vi "pulse data selector.vi"(0 "file path (dialog if empty)":path, 9 "y axis":u16(ring)=3 items=["time", "rate of change of B", "magnetic field", "signal A", "signal B", "1/B"]) -> (5 "file path":path, 6 "1/B start interpolation":dbl format="%.2f", 8 "1/B end interpolation":dbl format="%.2f", 10 "time rising":dbl[](array[numeric]) format="%.2f", 11 "ch B falling":dbl[](array[numeric]) format="%.2f", 12 "time falling":dbl[](array[numeric]) format="%.2f", 13 "ch B rising":dbl[](array[numeric]) format="%.2f", 14 "dB/dt rising":dbl[](array[numeric]) format="%.2f", 15 "dB/dt falling":dbl[](array[numeric]) format="%.2f", 16 "B rising":dbl[](array[numeric]) format="%.2f", 17 "B falling":dbl[](array[numeric]) format="%.2f", 18 "ch A rising":dbl[](array[numeric]) format="%.2f", 19 "ch A falling":dbl[](array[numeric]) format="%.2f")   [LabVIEW 2016]
uses:
  <vilib>/Utility/file.llb/Read From Spreadsheet File (DBL).vi
  <vilib>/Analysis/NI_AALPro.lvlib
panel:
  in  "subtract reference trace? copy 2":bool
  in  "mult fac.":dbl=1.0 format="%.2f"
  in  "subtract reference trace? copy":bool
  in  "with dB/dt":bool
  in  "background":u16(ring) items=["subtract fitted background", "divide the subtract 1"]
  in  "format":string="%f"
  in  "save plot?":bool
  in  "show":u16(ring) items=["rising and falling field", "rising field only", "falling field only"]
  in  "algorithm":u16(ring) items=["SVD", "Givens", "Givens2", "Householder", "LU Decomposition", "Cholesky"]
  out "?":u16(ring) items=["A"]
  in  "order":u8=1 step=1
  in  "subtract fitted background":u16(ring) items=["none", "polynomial in time", "polynomial in dB/dt", "polynomial in B", "polynomial in 1/B"]
  out "plotted data":cluster{dbl[], dbl[]}[](graph)
  in  "x axis":u16(ring)=2 items=["time", "rate of change of B", "magnetic field", "signal A", "signal B", "1/B"]
  in  "to":dbl=0.1 format="%.3f"
  in  "1/B from":dbl=0.01 format="%.3f"
  in  "to":dbl=70.0 format="%.2f"
  in  "B from":dbl format="%.2f"
  in  "special operation":u16(ring) items=["none", "renormalise by rate of field"]
  in  "selection":u16(ring) items=["all", "interval in field B", "interval in 1/B"]
  in  "to":u32=16384 min=1 step=1
  in  "from":u32=1 min=1 step=1
  in  "?":bool
  in  "subtract reference trace?":bool
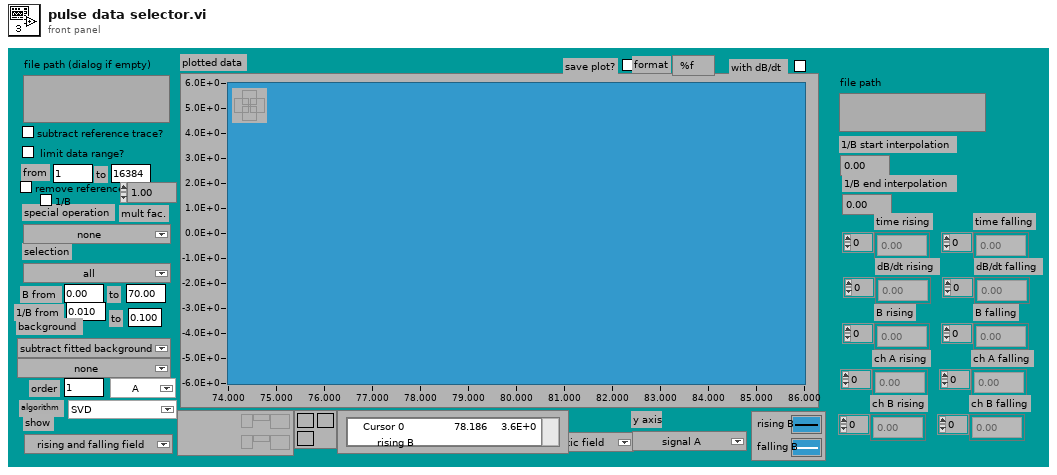
[diagram p1: front panel]
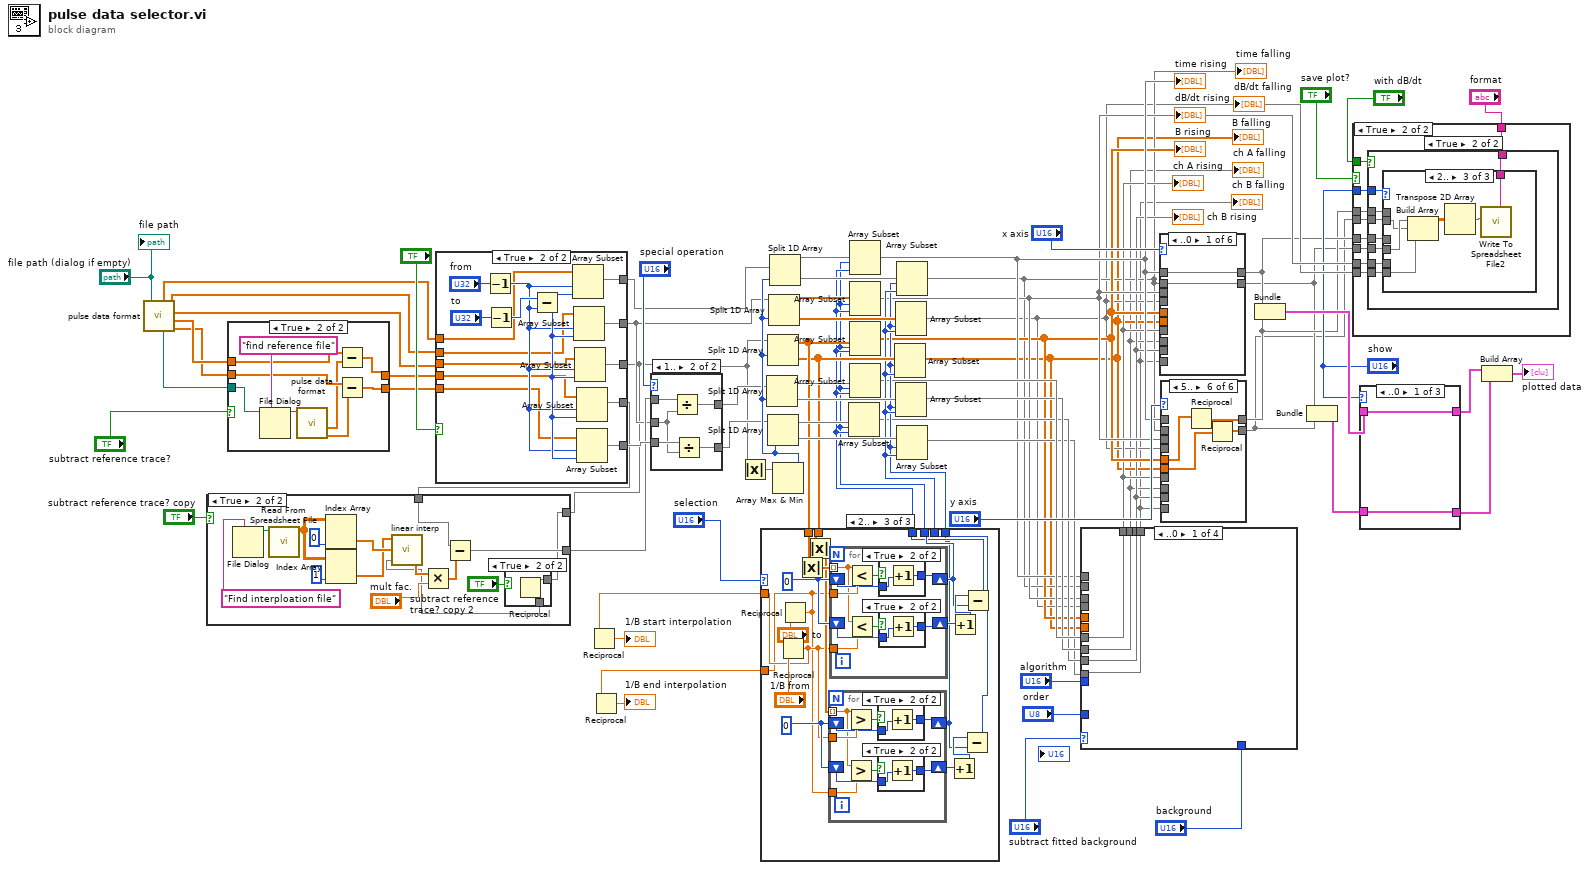
[diagram p0: block diagram]
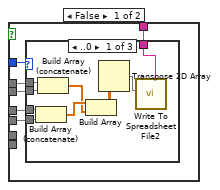
[diagram p5: hidden frame]
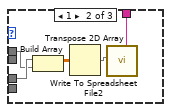
[diagram p6: hidden frame]
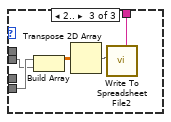
[diagram p7: hidden frame]
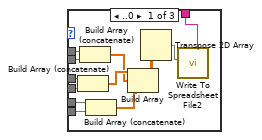
[diagram p8: hidden frame]
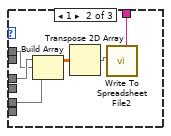
[diagram p9: hidden frame]
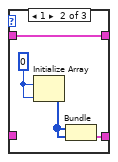
[diagram p10: hidden frame]
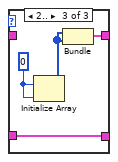
[diagram p11: hidden frame]
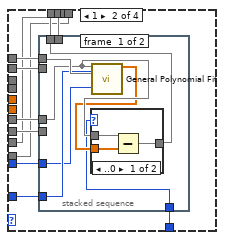
[diagram p12: hidden frame]
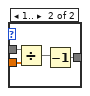
[diagram p13: hidden frame]
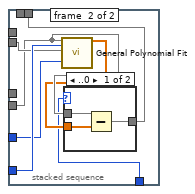
[diagram p14: hidden frame]
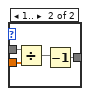
[diagram p15: hidden frame]
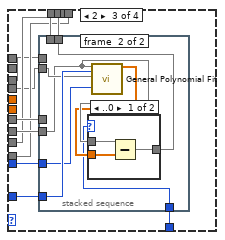
[diagram p16: hidden frame]
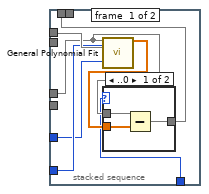
[diagram p17: hidden frame]
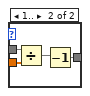
[diagram p18: hidden frame]
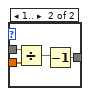
[diagram p19: hidden frame]
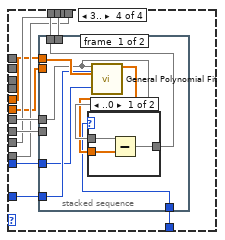
[diagram p20: hidden frame]
diagram:
  n1 = call "pulse data format.vi"("file path (dialog if empty)"="file path (dialog if empty)") -> ("time"=w70:dbl[], "file path read"=w72:path, "rate of change of field"=w69:dbl[], "magnetic field"=w68:dbl[], "signal channel A"=w74:dbl[], "signal channel B"=w73:dbl[])
  n2 = case shown="True" "subtract reference trace?" {
    tunnel: w74 -> [w77 w83]
    tunnel: w73 -> [w76 w82]
    tunnel: [w77 w79] -> w67
    tunnel: [w76 w78] -> w66
    tunnel: w72 -> [_ w86]
    frame False {
    }
    frame True {
      n3 = File Dialog(7:"find reference file", 11:w86) -> (3:w84:path)  [unwired: 5 in, 3 out]
      n4 = call "pulse data format.vi"("file path (dialog if empty)"=w84) -> ("signal channel A"=w81:dbl[], "signal channel B"=w80:dbl[])  [unwired: 4 out]
      n5 = Subtract(x=w83, y=w81) -> (x-y=w79:dbl[])
      n6 = Subtract(x=w82, y=w80) -> (x-y=w78:dbl[])
    }
  }
  n7 = case shown="True" "?" {
    tunnel: w70 -> [w91 w101]
    tunnel: w69 -> [w90 w100]
    tunnel: w68 -> [w89 w99]
    tunnel: w67 -> [w88 w98]
    tunnel: w66 -> [w87 w97]
    tunnel: [w91 w96] -> w58
    tunnel: [w90 w95] -> w2
    tunnel: [w88 w94] -> w5
    tunnel: [w87 w93] -> w64
    tunnel: [w89 w92] -> w1
    frame False {
    }
    frame True {
      n8 = Decrement(x="from") -> (x-1=w102:u32)
      n9 = Decrement(x="to") -> (x-1=w104:u32)
      n10 = Subtract(x=w104, y=w102) -> (x-y=w103:u32)
      n11 = Array Subset(array=w101, index=w102, length=w103) -> (w96:dbl[])
      n12 = Array Subset(array=w100, index=w102, length=w103) -> (w95:dbl[])
      n13 = Array Subset(array=w99, index=w102, length=w103) -> (w92:dbl[])
      n14 = Array Subset(array=w98, index=w102, length=w103) -> (w94:dbl[])
      n15 = Array Subset(array=w97, index=w102, length=w103) -> (w93:dbl[])
    }
  }
  n16 = case shown="True" "subtract reference trace? copy" {
    tunnel: w5 -> [w107 w117]
    tunnel: w1 -> [_ w110]
    tunnel: [w107 w116] -> w4
    frame False {
    }
    frame True {
      n17 = File Dialog(7:"Find interploation file") -> (3:w121:path)  [unwired: 6 in, 3 out]
      n18 = call-poly <vilib>:"Read From Spreadsheet File.vi"("file path (dialog if empty)"=w121) -> ("all rows"=w120:dbl[][])  [unwired: 6 in, 4 out]
      n19 = Index Array(array=w120, index (col)=0) -> (element=w119:dbl[])  [unwired: 1 in]
      n20 = Index Array(array=w120, index (col)=1) -> (element=w118:dbl[])  [unwired: 1 in]
      n21 = case shown="True" "subtract reference trace? copy 2" {
        tunnel: w110 -> [w123 w125]
        tunnel: [w123 w124] -> w108
        frame False {
        }
        frame True {
          n22 = Reciprocal(x=w125) -> (1/x=w124:dbl[])
        }
      }
      n23 = call "linear interp.vi"("x array"=w108, "X data"=w119, "Y data"=w118) -> ("y"=w115:dbl[])
      n24 = Multiply(x=w115, y="mult fac.") -> (x*y=w114:dbl[])
      n25 = Subtract(x=w117, y=w114) -> (x-y=w116:dbl[])
    }
  }
  n26 = case shown="1.." "special operation" {
    tunnel: w4 -> [w127 w132]
    tunnel: w64 -> [w126 w131]
    tunnel: w2 -> [_ w130]
    tunnel: [w126 w129] -> w56
    tunnel: [w127 w128] -> w57
    frame ..0 {
    }
    frame 1.. {
      n27 = Divide(x=w132, y=w130) -> (x/y=w128:dbl[])
      n28 = Divide(x=w131, y=w130) -> (x/y=w129:dbl[])
    }
  }
  n29 = Absolute Value(x=w1) -> (abs(x)=w63:dbl[])
  n30 = Array Max & Min(array=w63) -> (max index (indices)=w62:i32)  [unwired: 3 out]
  n31 = Split 1D Array(array=w57, index=w62) -> (first subarray=w52:dbl[], second subarray=w53:dbl[])
  n32 = Split 1D Array(array=w1, index=w62) -> (first subarray=w46:dbl[], second subarray=w45:dbl[])
  n33 = case shown="2.." "selection" {
    tunnel: w46 -> [w139 w155 w203]
    tunnel: w45 -> [w138 w149 w197]
    tunnel: [w137 w145 w193] -> w44
    tunnel: [w136 w142 w190] -> w43
    tunnel: [w135 w146 w194] -> w42
    tunnel: [w135 w143 w191] -> w41
    tunnel: [0.001 "B from" w186] -> w32
    tunnel: [100.0 "to" w187] -> w31
    frame ..0 {
      w135 = 0
      n34 = Array Size(array=w138) -> (size(s)=w136:i32)
      n35 = Array Size(array=w139) -> (size(s)=w137:i32)
    }
    frame 1 {
      w152 = 0
      w154 = 0
      n36 = Absolute Value(x=w155) -> (abs(x)=w150:dbl[])
      n37 = Absolute Value(x=w149) -> (abs(x)=w148:dbl[])
      n38 = for {
        tunnel: w148 -> [w158] mode=indexing
        shift-right: [w161] -> w143
        shift-left: w152 -> [w162]
        tunnel: "to" -> [w164]
        shift-right: [w156] -> w151
        shift-left: w152 -> [w159]
        tunnel: "B from" -> [w157]
        n39 = Greater?(x=w158, y=w164) -> (0:w163:bool)
        n40 = Greater?(x=w158, y=w157) -> (0:w160:bool)
        n41 = case shown="True" w163 {
          tunnel: w162 -> [w168 w169]
          tunnel: [w168 w170] -> w161
          frame False {
          }
          frame True {
            n42 = Increment(x=w169) -> (x+1=w170:i32)
          }
        }
        n43 = case shown="True" w160 {
          tunnel: w159 -> [w165 w166]
          tunnel: [w165 w167] -> w156
          frame False {
          }
          frame True {
            n44 = Increment(x=w166) -> (x+1=w167:i32)
          }
        }
      }
      n45 = for {
        tunnel: w150 -> [w173] mode=indexing
        shift-right: [w176] -> w146
        shift-left: w154 -> [w177]
        tunnel: "B from" -> [w179]
        shift-right: [w171] -> w153
        shift-left: w154 -> [w174]
        tunnel: "to" -> [w172]
        n46 = Less?(x=w173, y=w179) -> (x < y?=w178:bool)
        n47 = Less?(x=w173, y=w172) -> (x < y?=w175:bool)
        n48 = case shown="True" w178 {
          tunnel: w177 -> [w183 w184]
          tunnel: [w183 w185] -> w176
          frame False {
          }
          frame True {
            n49 = Increment(x=w184) -> (x+1=w185:i32)
          }
        }
        n50 = case shown="True" w175 {
          tunnel: w174 -> [w180 w181]
          tunnel: [w180 w182] -> w171
          frame False {
          }
          frame True {
            n51 = Increment(x=w181) -> (x+1=w182:i32)
          }
        }
      }
      n52 = Increment(x=w151) -> (x+1=w144:i32)
      n53 = Increment(x=w153) -> (x+1=w147:i32)
      n54 = Subtract(x=w144, y=w143) -> (x-y=w142:i32)
      n55 = Subtract(x=w147, y=w146) -> (x-y=w145:i32)
    }
    frame 2.. {
      w200 = 0
      w202 = 0
      n56 = Reciprocal(x="1/B from") -> (1/x=w187:dbl)
      n57 = Reciprocal(x="to") -> (1/x=w186:dbl)
      n58 = Absolute Value(x=w203) -> (abs(x)=w198:dbl[])
      n59 = Absolute Value(x=w197) -> (abs(x)=w196:dbl[])
      n60 = for {
        tunnel: w196 -> [w206] mode=indexing
        shift-right: [w209] -> w191
        shift-left: w200 -> [w210]
        tunnel: w187 -> [w212]
        shift-right: [w204] -> w199
        shift-left: w200 -> [w207]
        tunnel: w186 -> [w205]
        n61 = Greater?(x=w206, y=w212) -> (0:w211:bool)
        n62 = Greater?(x=w206, y=w205) -> (0:w208:bool)
        n63 = case shown="True" w211 {
          tunnel: w210 -> [w216 w217]
          tunnel: [w216 w218] -> w209
          frame False {
          }
          frame True {
            n64 = Increment(x=w217) -> (x+1=w218:i32)
          }
        }
        n65 = case shown="True" w208 {
          tunnel: w207 -> [w213 w214]
          tunnel: [w213 w215] -> w204
          frame False {
          }
          frame True {
            n66 = Increment(x=w214) -> (x+1=w215:i32)
          }
        }
      }
      n67 = for {
        tunnel: w198 -> [w221] mode=indexing
        shift-right: [w224] -> w194
        shift-left: w202 -> [w225]
        tunnel: w186 -> [w227]
        shift-right: [w219] -> w201
        shift-left: w202 -> [w222]
        tunnel: w187 -> [w220]
        n68 = Less?(x=w221, y=w227) -> (x < y?=w226:bool)
        n69 = Less?(x=w221, y=w220) -> (x < y?=w223:bool)
        n70 = case shown="True" w226 {
          tunnel: w225 -> [w231 w232]
          tunnel: [w231 w233] -> w224
          frame False {
          }
          frame True {
            n71 = Increment(x=w232) -> (x+1=w233:i32)
          }
        }
        n72 = case shown="True" w223 {
          tunnel: w222 -> [w228 w229]
          tunnel: [w228 w230] -> w219
          frame False {
          }
          frame True {
            n73 = Increment(x=w229) -> (x+1=w230:i32)
          }
        }
      }
      n74 = Increment(x=w199) -> (x+1=w192:i32)
      n75 = Increment(x=w201) -> (x+1=w195:i32)
      n76 = Subtract(x=w192, y=w191) -> (x-y=w190:i32)
      n77 = Subtract(x=w195, y=w194) -> (x-y=w193:i32)
    }
  }
  n78 = Reciprocal(x=w31) -> (1/x=→"1/B start interpolation":dbl)
  n79 = Reciprocal(x=w32) -> (1/x=→"1/B end interpolation":dbl)
  n80 = Split 1D Array(array=w56, index=w62) -> (first subarray=w54:dbl[], second subarray=w55:dbl[])
  n81 = Split 1D Array(array=w2, index=w62) -> (first subarray=w50:dbl[], second subarray=w51:dbl[])
  n82 = Split 1D Array(array=w58, index=w62) -> (first subarray=w48:dbl[], second subarray=w49:dbl[])
  n83 = Array Subset(array=w54, index=w42, length=w44) -> (w37:dbl[])
  n84 = Array Subset(array=w48, index=w42, length=w44) -> (w26:dbl[])
  "time rising" <- w26
  n85 = Array Subset(array=w50, index=w42, length=w44) -> (w25:dbl[])
  "dB/dt rising" <- w25
  n86 = Array Subset(array=w46, index=w42, length=w44) -> (w24:dbl[])
  "B rising" <- w24
  n87 = Array Subset(array=w52, index=w42, length=w44) -> (w39:dbl[])
  n88 = Array Subset(array=w45, index=w41, length=w43) -> (w19:dbl[])
  "B falling" <- w19
  n89 = Array Subset(array=w51, index=w41, length=w43) -> (w20:dbl[])
  "dB/dt falling" <- w20
  n90 = Array Subset(array=w53, index=w41, length=w43) -> (w38:dbl[])
  n91 = Array Subset(array=w49, index=w41, length=w43) -> (w21:dbl[])
  "time falling" <- w21
  n92 = Array Subset(array=w55, index=w41, length=w43) -> (w36:dbl[])
  n93 = case shown="..0" "subtract fitted background" {
    tunnel: w26 -> [_ w248 _ _]
    tunnel: w21 -> [_ w247 _ _]
    tunnel: w25 -> [_ _ w279 _]
    tunnel: w20 -> [_ _ w278 _]
    tunnel: w24 -> [_ _ _ w318]
    tunnel: w19 -> [_ _ _ w317]
    tunnel: w39 -> [w237 w246 w287 w326]
    tunnel: w38 -> [w236 w245 w286 w325]
    tunnel: w37 -> [w235 w240 w281 w320]
    tunnel: w36 -> [w234 w239 w280 w319]
    tunnel: [w237 w242 w283 w322] -> w23
    tunnel: [w236 w241 w282 w321] -> w18
    tunnel: [w235 w240 w281 w320] -> w22
    tunnel: [w234 w239 w280 w319] -> w17
    tunnel: "order" -> [_ w244 w285 w324]
    tunnel: "algorithm" -> [_ w243 w284 w323]
    tunnel: "background" -> [_ w238 w277 w316]
    frame ..0 {
    }
    frame 1 {
      n94 = stacked-sequence {
        tunnel: w248 -> [w255 _]
        tunnel: w247 -> [_ w267]
        tunnel: w246 -> [w252 _]
        tunnel: w245 -> [_ w266]
        tunnel: w244 -> [w254 w269]
        tunnel: w243 -> [w253 w268]
        tunnel: [w250 _] -> w242
        tunnel: [_ w264] -> w241
        tunnel: w238 -> [w249 w263]
        frame #0 {
          n95 = call <vilib>:"General Polynomial Fit.vi"("Y"=w252, "polynomial order"=w254, "X"=w255, "algorithm"=w253) -> ("Best Polynomial Fit"=w251:dbl[])  [unwired: 8 in, 3 out]
          n96 = case shown="..0" w249 {
            tunnel: w252 -> [w258 w262]
            tunnel: w251 -> [w257 w261]
            tunnel: [w256 w259] -> w250
            frame ..0 {
              n97 = Subtract(x=w258, y=w257) -> (x-y=w256:dbl[])
            }
            frame 1.. {
              n98 = Divide(x=w262, y=w261) -> (x/y=w260:dbl[])
              n99 = Decrement(x=w260) -> (x-1=w259:dbl[])
            }
          }
        }
        frame #1 {
          n100 = call <vilib>:"General Polynomial Fit.vi"("Y"=w266, "polynomial order"=w269, "X"=w267, "algorithm"=w268) -> ("Best Polynomial Fit"=w265:dbl[])  [unwired: 8 in, 3 out]
          n101 = case shown="..0" w263 {
            tunnel: w266 -> [w272 w276]
            tunnel: w265 -> [w271 w275]
            tunnel: [w270 w273] -> w264
            frame ..0 {
              n102 = Subtract(x=w272, y=w271) -> (x-y=w270:dbl[])
            }
            frame 1.. {
              n103 = Divide(x=w276, y=w275) -> (x/y=w274:dbl[])
              n104 = Decrement(x=w274) -> (x-1=w273:dbl[])
            }
          }
        }
      }
    }
    frame 2 {
      n105 = stacked-sequence {
        tunnel: w279 -> [w294 _]
        tunnel: w278 -> [_ w306]
        tunnel: w287 -> [w291 _]
        tunnel: w286 -> [_ w305]
        tunnel: w285 -> [w293 w308]
        tunnel: w284 -> [w292 w307]
        tunnel: [w288 _] -> w283
        tunnel: [_ w303] -> w282
        tunnel: w277 -> [w289 w302]
        frame #0 {
          n106 = call <vilib>:"General Polynomial Fit.vi"("Y"=w291, "polynomial order"=w293, "X"=w294, "algorithm"=w292) -> ("Best Polynomial Fit"=w290:dbl[])  [unwired: 8 in, 3 out]
          n107 = case shown="..0" w289 {
            tunnel: w291 -> [w297 w301]
            tunnel: w290 -> [w296 w300]
            tunnel: [w295 w298] -> w288
            frame ..0 {
              n108 = Subtract(x=w297, y=w296) -> (x-y=w295:dbl[])
            }
            frame 1.. {
              n109 = Divide(x=w301, y=w300) -> (x/y=w299:dbl[])
              n110 = Decrement(x=w299) -> (x-1=w298:dbl[])
            }
          }
        }
        frame #1 {
          n111 = call <vilib>:"General Polynomial Fit.vi"("Y"=w305, "polynomial order"=w308, "X"=w306, "algorithm"=w307) -> ("Best Polynomial Fit"=w304:dbl[])  [unwired: 8 in, 3 out]
          n112 = case shown="..0" w302 {
            tunnel: w305 -> [w311 w315]
            tunnel: w304 -> [w310 w314]
            tunnel: [w309 w312] -> w303
            frame ..0 {
              n113 = Subtract(x=w311, y=w310) -> (x-y=w309:dbl[])
            }
            frame 1.. {
              n114 = Divide(x=w315, y=w314) -> (x/y=w313:dbl[])
              n115 = Decrement(x=w313) -> (x-1=w312:dbl[])
            }
          }
        }
      }
    }
    frame 3.. {
      n116 = stacked-sequence {
        tunnel: w318 -> [w333 _]
        tunnel: w317 -> [_ w345]
        tunnel: w326 -> [w330 _]
        tunnel: w325 -> [_ w343]
        tunnel: w324 -> [w332 w347]
        tunnel: w323 -> [w331 w346]
        tunnel: [w327 _] -> w322
        tunnel: [_ w341] -> w321
        tunnel: w316 -> [w328 w344]
        frame #0 {
          n117 = call <vilib>:"General Polynomial Fit.vi"("Y"=w330, "polynomial order"=w332, "X"=w333, "algorithm"=w331) -> ("Best Polynomial Fit"=w329:dbl[])  [unwired: 8 in, 3 out]
          n118 = case shown="..0" w328 {
            tunnel: w330 -> [w336 w340]
            tunnel: w329 -> [w335 w339]
            tunnel: [w334 w337] -> w327
            frame ..0 {
              n119 = Subtract(x=w336, y=w335) -> (x-y=w334:dbl[])
            }
            frame 1.. {
              n120 = Divide(x=w340, y=w339) -> (x/y=w338:dbl[])
              n121 = Decrement(x=w338) -> (x-1=w337:dbl[])
            }
          }
        }
        frame #1 {
          n122 = call <vilib>:"General Polynomial Fit.vi"("Y"=w343, "polynomial order"=w347, "X"=w345, "algorithm"=w346) -> ("Best Polynomial Fit"=w342:dbl[])  [unwired: 8 in, 3 out]
          n123 = case shown="..0" w344 {
            tunnel: w343 -> [w350 w354]
            tunnel: w342 -> [w349 w353]
            tunnel: [w348 w351] -> w341
            frame ..0 {
              n124 = Subtract(x=w350, y=w349) -> (x-y=w348:dbl[])
            }
            frame 1.. {
              n125 = Divide(x=w354, y=w353) -> (x/y=w352:dbl[])
              n126 = Decrement(x=w352) -> (x-1=w351:dbl[])
            }
          }
        }
      }
    }
  }
  "ch A rising" <- w23
  "ch B rising" <- w22
  "ch A falling" <- w18
  "ch B falling" <- w17
  n127 = case shown="..0" "x axis" {
    tunnel: w26 -> [w356 _ _ _ _ _]
    tunnel: w21 -> [w355 _ _ _ _ _]
    tunnel: w25 -> [_ w358 _ _ _ _]
    tunnel: w20 -> [_ w357 _ _ _ _]
    tunnel: w24 -> [_ _ w360 _ _ w366]
    tunnel: w19 -> [_ _ w359 _ _ w365]
    tunnel: w23 -> [_ _ _ w362 _ _]
    tunnel: w18 -> [_ _ _ w361 _ _]
    tunnel: w22 -> [_ _ _ _ w364 _]
    tunnel: w17 -> [_ _ _ _ w363 _]
    tunnel: [w356 w358 w360 w362 w364 w367] -> w14
    tunnel: [w355 w357 w359 w361 w363 w368] -> w12
    frame ..0 {
    }
    frame 1 {
    }
    frame 2 {
    }
    frame 3 {
    }
    frame 4 {
    }
    frame 5.. {
      n128 = Reciprocal(x=w366) -> (1/x=w367:dbl[])
      n129 = Reciprocal(x=w365) -> (1/x=w368:dbl[])
    }
  }
  n130 = case shown="5.." "y axis" {
    tunnel: w26 -> [w370 _ _ _ _ _]
    tunnel: w21 -> [w369 _ _ _ _ _]
    tunnel: w25 -> [_ w372 _ _ _ _]
    tunnel: w20 -> [_ w371 _ _ _ _]
    tunnel: w24 -> [_ _ w374 _ _ w380]
    tunnel: w19 -> [_ _ w373 _ _ w379]
    tunnel: w23 -> [_ _ _ w376 _ _]
    tunnel: w18 -> [_ _ _ w375 _ _]
    tunnel: w22 -> [_ _ _ _ w378 _]
    tunnel: w17 -> [_ _ _ _ w377 _]
    tunnel: [w370 w372 w374 w376 w378 w382] -> w13
    tunnel: [w369 w371 w373 w375 w377 w381] -> w11
    frame ..0 {
    }
    frame 1 {
    }
    frame 2 {
    }
    frame 3 {
    }
    frame 4 {
    }
    frame 5.. {
      n131 = Reciprocal(x=w380) -> (1/x=w382:dbl[])
      n132 = Reciprocal(x=w379) -> (1/x=w381:dbl[])
    }
  }
  n133 = Bundle(w14, w13) -> (w29:cluster{dbl[], dbl[]})  [unwired: 1 in]
  n134 = Bundle(w12, w11) -> (w27:cluster{dbl[], dbl[]})  [unwired: 1 in]
  n135 = case shown="True" "save plot?" {
    tunnel: "show" -> [_ w385]
    tunnel: w14 -> [_ w388]
    tunnel: w12 -> [_ w387]
    tunnel: w13 -> [_ w390]
    tunnel: w11 -> [_ w389]
    tunnel: "format" -> [_ w386]
    tunnel: "with dB/dt" -> [_ w391]
    tunnel: w25 -> [_ w384]
    tunnel: w20 -> [_ w383]
    frame False {
    }
    frame True {
      n136 = case shown="True" w391 {
        tunnel: w390 -> [w397 w424]
        tunnel: w389 -> [w396 w423]
        tunnel: w388 -> [w395 w422]
        tunnel: w387 -> [w394 w421]
        tunnel: w386 -> [w393 w420]
        tunnel: w385 -> [w392 w419]
        tunnel: w384 -> [_ w418]
        tunnel: w383 -> [_ w417]
        frame False {
          n137 = case shown="..0" w392 {
            tunnel: w395 -> [w406 w408 _]
            tunnel: w394 -> [w405 _ w413]
            tunnel: w397 -> [w404 w407 _]
            tunnel: w396 -> [w403 _ w412]
            tunnel: w393 -> [w401 w409 w415]
            frame ..0 {
              n138 = Build Array (concatenate)(w406, w405) -> (w399:dbl[])
              n139 = Build Array (concatenate)(w404, w403) -> (w398:dbl[])
              n140 = Build Array(w399, w398) -> (w402:dbl[][])
              n141 = Transpose 2D Array(2D array=w402) -> (transposed array=w400:dbl[][])
              n142 = call "Write To Spreadsheet File2.vi"("format (%.3f)"=w401, "2D data"=w400) -> ()  [unwired: 6 in, 1 out]
            }
            frame 1 {
              n143 = Build Array(w408, w407) -> (w411:dbl[][])
              n144 = Transpose 2D Array(2D array=w411) -> (transposed array=w410:dbl[][])
              n145 = call "Write To Spreadsheet File2.vi"("format (%.3f)"=w409, "2D data"=w410) -> ()  [unwired: 6 in, 1 out]
            }
            frame 2.. {
              n146 = Build Array(w413, w412) -> (w416:dbl[][])
              n147 = Transpose 2D Array(2D array=w416) -> (transposed array=w414:dbl[][])
              n148 = call "Write To Spreadsheet File2.vi"("format (%.3f)"=w415, "2D data"=w414) -> ()  [unwired: 6 in, 1 out]
            }
          }
        }
        frame True {
          n149 = case shown="2.." w419 {
            tunnel: w422 -> [w436 w439 _]
            tunnel: w421 -> [w435 _ w445]
            tunnel: w424 -> [w434 w438 _]
            tunnel: w423 -> [w433 _ w444]
            tunnel: w420 -> [w431 w440 w447]
            tunnel: w418 -> [w427 w437 _]
            tunnel: w417 -> [w426 _ w443]
            frame ..0 {
              n150 = Build Array (concatenate)(w436, w435) -> (w429:dbl[])
              n151 = Build Array (concatenate)(w434, w433) -> (w428:dbl[])
              n152 = Build Array (concatenate)(w427, w426) -> (w425:dbl[])
              n153 = Build Array(w429, w428, w425) -> (w432:dbl[][])
              n154 = Transpose 2D Array(2D array=w432) -> (transposed array=w430:dbl[][])
              n155 = call "Write To Spreadsheet File2.vi"("format (%.3f)"=w431, "2D data"=w430) -> ()  [unwired: 6 in, 1 out]
            }
            frame 1 {
              n156 = Build Array(w439, w438, w437) -> (w442:dbl[][])
              n157 = Transpose 2D Array(2D array=w442) -> (transposed array=w441:dbl[][])
              n158 = call "Write To Spreadsheet File2.vi"("format (%.3f)"=w440, "2D data"=w441) -> ()  [unwired: 6 in, 1 out]
            }
            frame 2.. {
              n159 = Build Array(w445, w444, w443) -> (w448:dbl[][])
              n160 = Transpose 2D Array(2D array=w448) -> (transposed array=w446:dbl[][])
              n161 = call "Write To Spreadsheet File2.vi"("format (%.3f)"=w447, "2D data"=w446) -> ()  [unwired: 6 in, 1 out]
            }
          }
        }
      }
    }
  }
  n162 = case shown="..0" "show" {
    tunnel: [w450 w454 w455] -> w30
    tunnel: w29 -> [w450 w454 _]
    tunnel: [w449 w451 w456] -> w28
    tunnel: w27 -> [w449 _ w456]
    frame ..0 {
    }
    frame 1 {
      w453 = 0
      n163 = Initialize Array(w453, w453) -> (w452:i32[])
      n164 = Bundle(w452, w452) -> (w451:cluster{i32[], i32[]})  [unwired: 1 in]
    }
    frame 2.. {
      w458 = 0
      n165 = Initialize Array(w458, w458) -> (w457:i32[])
      n166 = Bundle(w457, w457) -> (w455:cluster{i32[], i32[]})  [unwired: 1 in]
    }
  }
  n167 = Build Array(w30, w28) -> (→"plotted data":cluster{dbl[], dbl[]}[])
  "file path" <- "file path (dialog if empty)"
